vi "例程16-产生两个函数曲线.vi"() -> ()   [LabVIEW 2016]
panel:
  out "XY Graph":cluster{"Y":dbl[], "Y":dbl[]}[](graph)=[{"Y"=[0.0, 1.0, 2.0, 3.0, 4.0, 5.0, 6.0, 7.0, 8.0, 9.0, 10.0, 11.0, 12.0, 13.0, 14.0, 15.0, 16.0, 17.0, 18.0, 19.0], "Y"=[100.0, 110.00000000000001, 120.0, 130.0, 140.0, 150.0, 160.0, 170.00000000000003, 180.0, 190.0, 200.0, 210.0, 220.00000000000003, 229.99999999999997, 240.00000000000003, 250.0, 260.0, 270.0, 280.0, 290.00000000000006]}, {"Y"=[0.0, 1.0, 2.0, 3.0, 4.0, 5.0, 6.0, 7.0, 8.0, 9.0, 10.0, 11.0, 12.0, 13.0, 14.0, 15.0, 16.0, 17.0, 18.0, 19.0], "Y"=[100.0, 110.00000000000001, 121.00000000000001, 133.10000000000005, 146.41000000000005, 161.05100000000004, 177.1561000000001, 194.87171000000012, 214.35888100000017, 235.7947691000002, 259.3742460100002, 285.31167061100024, 313.8428376721003, 345.2271214393104, 379.7498335832414, 417.7248169415656, 459.4972986357222, 505.4470284992945, 555.991731349224, 611.5909044841464]}] caption="XY图"
  in  "Y":dbl=0.1
  in  "X":dbl=100.0
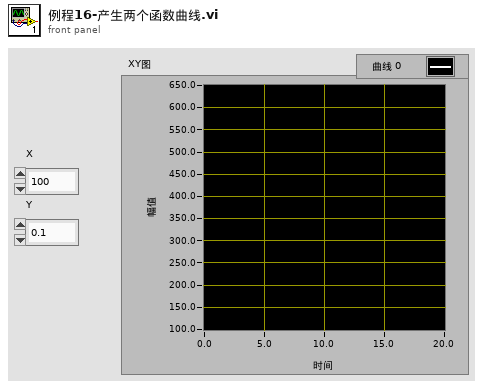
[diagram p1: front panel]
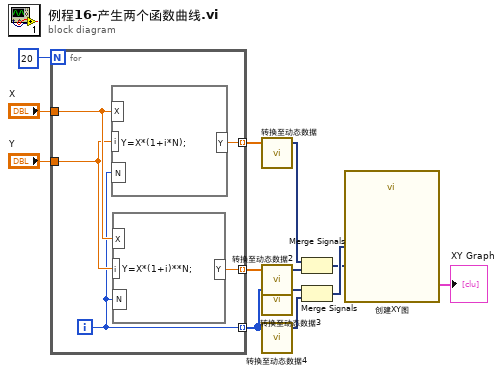
[diagram p0: block diagram]
diagram:
  n1 = for {
    N: 20 -> [_]
    tunnel: "X" -> [w18]
    tunnel: "Y" -> [w17]
    tunnel: [w16] -> w10 mode=indexing
    tunnel: [w15] -> w9 mode=indexing
    tunnel: [w14] -> w8 mode=indexing
    i -> [w14]
    n2 = formula code="Y=X*(1+i*N);"("X"=w18, "i"=w17, "N"=w14) -> ("Y"=w15:dbl)
    n3 = formula code="Y=X*(1+i)**N;"("X"=w18, "i"=w17, "N"=w14) -> ("Y"=w16:dbl)
  }
  n4 = call "转换至动态数据"("Array"=w9) -> ("Dynamic Data Type"=w7:dynamicdata)  [unwired: 3 in]
  n5 = call "转换至动态数据2"("Array"=w10) -> ("Dynamic Data Type"=w6:dynamicdata)  [unwired: 3 in]
  n6 = call "转换至动态数据3"("Array"=w8) -> ("Dynamic Data Type"=w5:dynamicdata)  [unwired: 3 in]
  n7 = call "转换至动态数据4"("Array"=w8) -> ("Dynamic Data Type"=w4:dynamicdata)  [unwired: 3 in]
  n8 = Merge Signals(w7, w6) -> (w1:dynamicdata)
  n9 = Merge Signals(w5, w4) -> (w2:dynamicdata)
  n10 = call "创建XY图"("Y Input"=w1, "X Input"=w2) -> ("XY Graph"=→"XY Graph":cluster{"X":dbl[], "Y":dbl[]}[])  [unwired: 8 in, 1 out]
